vi "Decode_sequence_file.vi"(6 "error in":errorcluster, 9 "file (use dialog)":path) -> (0 "error out":errorcluster, 1 "Waveform Filenames":string[][](array[string]), 2 "Number of lines":i32, 3 "Number of channels":i32, 4 "Sample Clock":dbl, 5 "text":string)   [LabVIEW 2010]
panel:
  out "Array":string[](array[string])
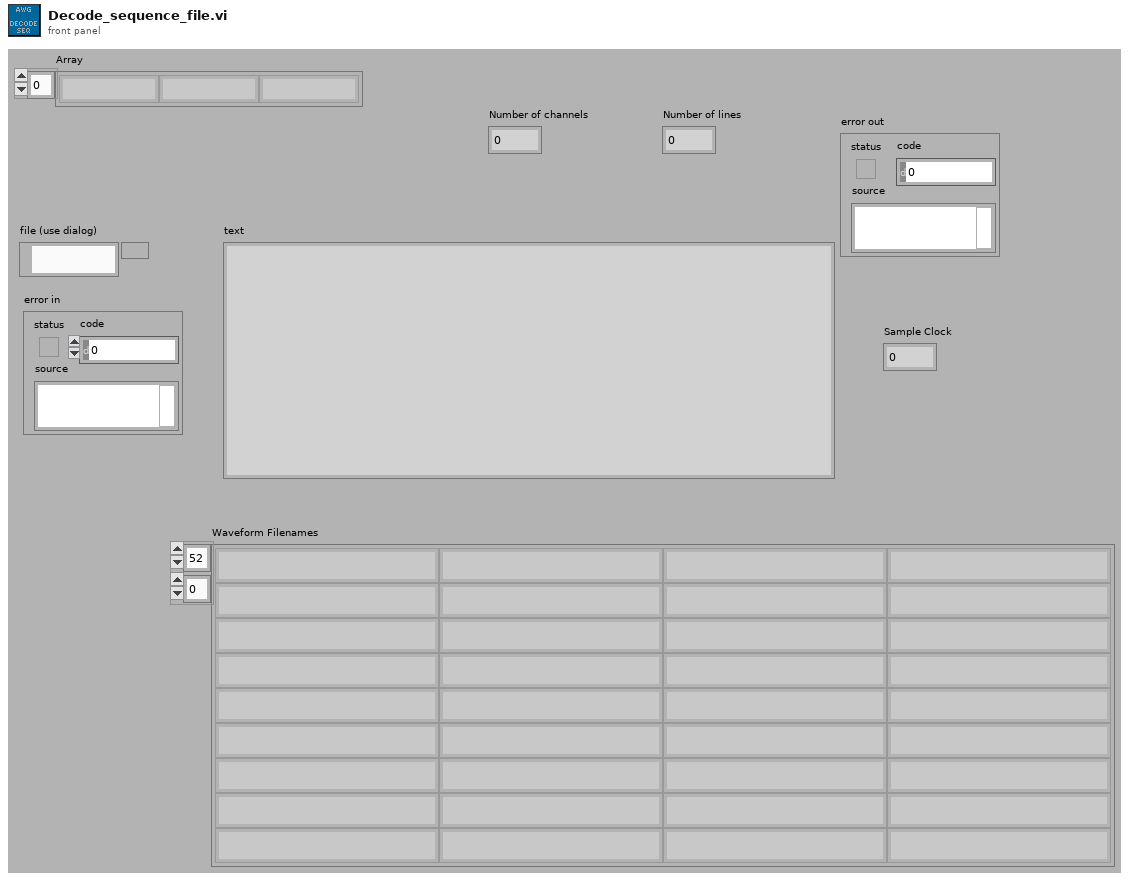
[diagram p1: front panel]
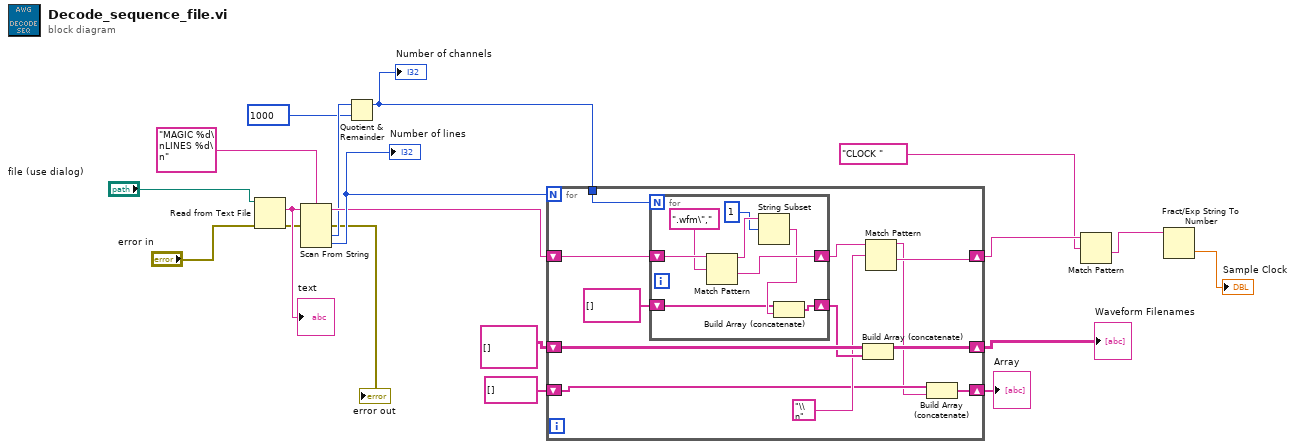
[diagram p0: block diagram]
diagram:
  n1 = Read from Text File(file (use dialog)="file (use dialog)", error in="error in") -> (text=w16:string, error out=→"error out":errorcluster)  [unwired: 2 in, 2 out]
  "text" <- w16
  n2 = Scan From String(format string="MAGIC %d\nLINES %d\n", input string=w16) -> (remaining string=w13:string, output 1=w12:i32, output 2=w14:i32)  [unwired: 4 in, 2 out]
  "Number of lines" <- w14
  n3 = Quotient & Remainder(x=w12, y=1000) -> (x-y*floor(x/y)=w9:i32)  [unwired: 1 out]
  "Number of channels" <- w9
  n4 = for {
    N: w14 -> [_]
    shift-right: [w29] -> w8
    shift-left: string[][] [] -> [w28]
    shift-right: [w22] -> w6
    shift-left: w13 -> [w30]
    tunnel: w9 -> [w27]
    shift-right: [w21] -> w1
    shift-left: string[] [] -> [w20]
    n5 = for {
      N: w27 -> [_]
      shift-right: [w36] -> w24
      shift-left: w30 -> [w38]
      shift-right: [w32] -> w25
      shift-left: string[] [] -> [w31]
      n6 = Match Pattern(string=w38, regular expression=".wfm\"," ("format string")) -> (before substring=w35:string, after substring=w36:string)  [unwired: 1 in, 2 out]
      n7 = String Subset(string=w35, offset (0)=1) -> (substring=w33:string)  [unwired: 1 in]
      n8 = Build Array (concatenate)(w31, w33) -> (w32:string[])
    }
    n9 = Build Array (concatenate)(w28, w25) -> (w29:string[][])
    n10 = Match Pattern(string=w24, regular expression="\\n") -> (before substring=w19:string, after substring=w22:string)  [unwired: 1 in, 2 out]
    n11 = Build Array (concatenate)(w20, w19) -> (w21:string[])
  }
  "Waveform Filenames" <- w8
  "Array" <- w1
  n12 = Match Pattern(string=w6, regular expression="CLOCK " ("format string")) -> (after substring=w4:string)  [unwired: 1 in, 3 out]
  n13 = Fract/Exp String To Number(string=w4) -> (number=→"Sample Clock":dbl)  [unwired: 3 in, 1 out]
